vi "Configure Trigger (Pattern).vi"(0 "VISA resource name":refnum<visa-resource-name>, 1 "Pattern Mask (0)":u16, 2 "Edge Source (0: None)":u16(ring) items=["Channel 1"=0, "Channel 2"=1, "Channel 3"=2, "Channel 4"=3, "EXT5"=5, "Digital 0"=7, "Digital 1"=8, "Digital 2"=9, "Digital 3"=10, "Digital 4"=11, "Digital 5"=12, "Digital 6"=13, "Digital 7"=14, "Digital 8"=15, "Digital 9"=16, "Digital 10"=17, "Digital 11"=18, "Digital 12"=19, "Digital 13"=20, "Digital 14"=21, "Digital 15"=22], 3 "Configure Edge (Disable)":bool, 5 "Trigger Source (0: Channel 1)":i32(ring) items=["Channel 1", "Channel 2", "Channel 3", "Channel 4", "EXT", "EXT5", "AC Line", "Digital 0", "Digital 1", "Digital 2", "Digital 3", "Digital 4", "Digital 5", "Digital 6", "Digital 7", "Digital 8", "Digital 9", "Digital 10", "Digital 11", "Digital 12", "Digital 13", "Digital 14", "Digital 15"], 7 "Trigger Level (0.0 V)":dbl, 9 "Pattern Value (0)":u16, 11 "error in (no error)":errorcluster, 12 "EXT Source (0: EXT)":u16(ring) items=["EXT", "EXT5"], 13 "Edge (0: None)":u16(ring) items=["Positive", "Negative"]) -> (4 "VISA resource name out":refnum<visa-resource-name>, 15 "error out":errorcluster)   [LabVIEW 2012, in "RIGOL DS1000 Series.lvlib"]
doc: "Configures pattern trigger settings for an oscilloscope.\n\n<b>Note:</b>\n\nThis VI only applies to the Rigol DS1000B and DS1000D Series models."
uses:
  RIGOL DS1000 Series.lvlib
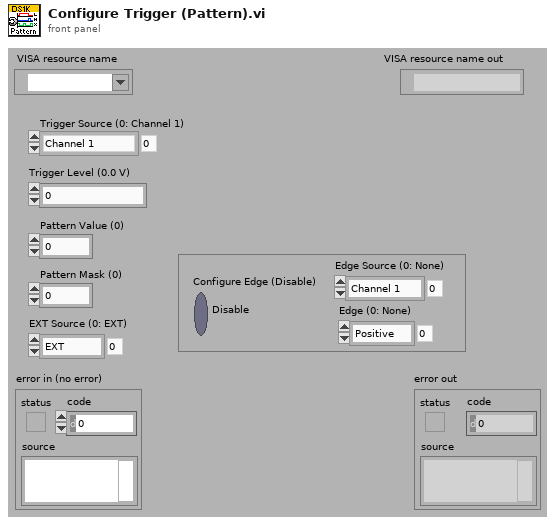
[diagram p1: front panel]
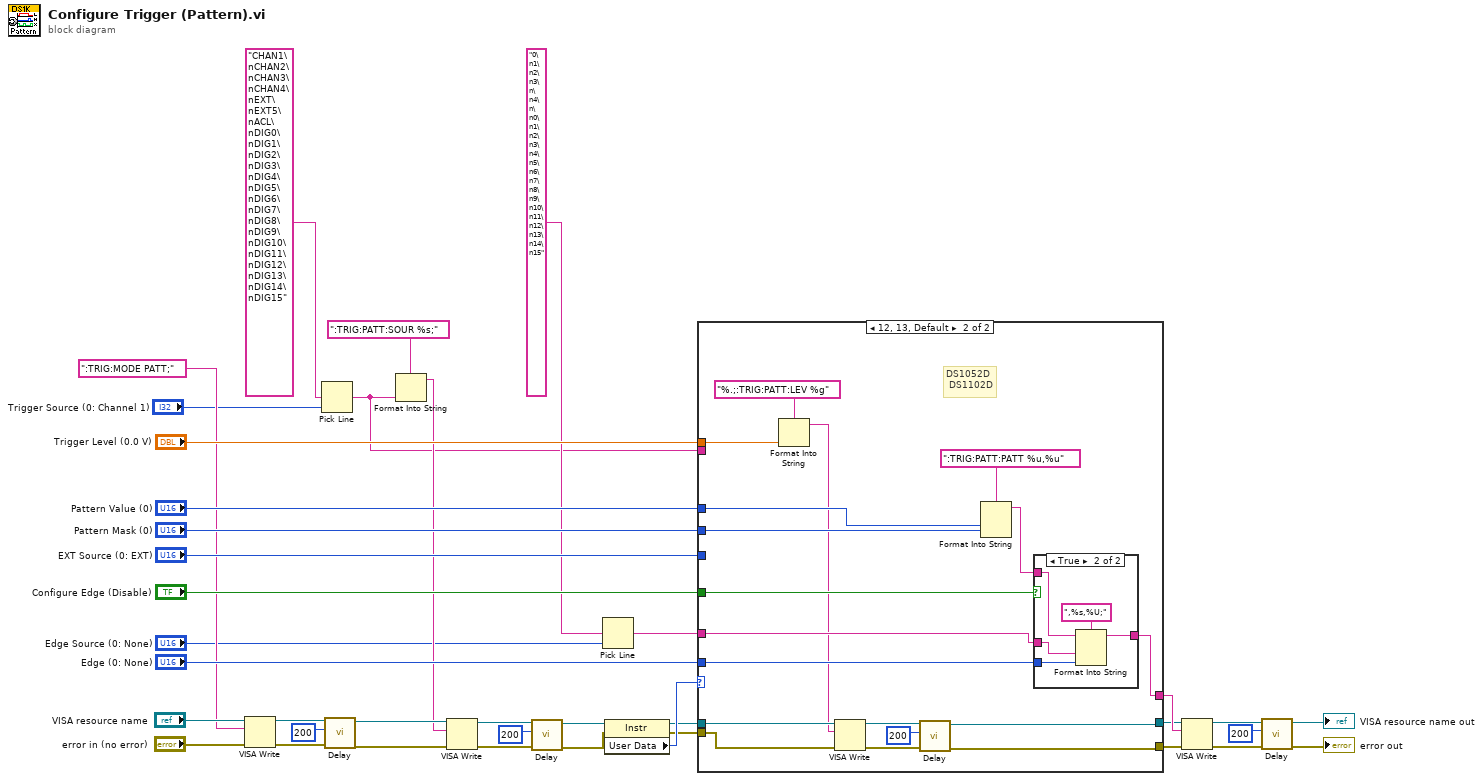
[diagram p0: block diagram]
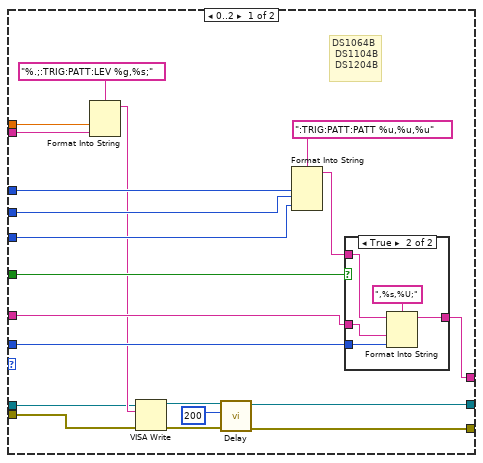
[diagram p2: hidden frame]
diagram:
  n1 = VISA Write(VISA resource name="VISA resource name", write buffer=":TRIG:MODE PATT;" ("Pattern Trigger Type"), error in (no error)="error in (no error)") -> (VISA resource name out=w23:refnum<visa-resource-name>, error out=w24:errorcluster)  [unwired: 1 out]
  n2 = Pick Line(multi-line string="CHAN1\nCHAN2\nCHAN3\nCHAN4\nEXT\nEXT5\nACL\nDIG0\nDIG1\nDIG2\nDIG3\nDIG4\nDIG5\nDIG6\nDIG7\nDIG8\nDIG9\nDIG10\nDIG11\nDIG12\nDIG13\nDIG14\nDIG15" ("多行字符串"), line index="Trigger Source (0: Channel 1)") -> (output string=w1:string)  [unwired: 1 out]
  n3 = call "Delay.vi"("error in (no error)"=w24, "Delay (ms)"=u32 200, "VISA resource name"=w23) -> ("error out"=w14:errorcluster, "VISA resource name out"=w15:refnum<visa-resource-name>)  [unwired: 7 out]
  n4 = Format Into String(format string=":TRIG:PATT:SOUR %s;", w1) -> (resulting string=w13:string)  [unwired: 2 in, 1 out]
  n5 = VISA Write(VISA resource name=w15, write buffer=w13, error in (no error)=w14) -> (VISA resource name out=w17:refnum<visa-resource-name>, error out=w18:errorcluster)  [unwired: 1 out]
  n6 = call "Delay.vi"("error in (no error)"=w18, "Delay (ms)"=u32 200, "VISA resource name"=w17) -> ("error out"=w7:errorcluster, "VISA resource name out"=w8:refnum<visa-resource-name>)  [unwired: 7 out]
  n7 = Pick Line(multi-line string="0\n1\n2\n3\n\n4\n\n0\n1\n2\n3\n4\n5\n6\n7\n8\n9\n10\n11\n12\n13\n14\n15" ("多行字符串"), line index="Edge Source (0: None)") -> (output string=w9:string)  [unwired: 1 out]
  n8 = property class="Instr"(reference=w8, error in=w7) -> (reference out=w5:refnum<visa-resource-name>, error out=w4:errorcluster, "User Data"=w6:u32)
  n9 = case shown="12, 13, Default" w6 {
    tunnel: "Trigger Level (0.0 V)" -> [w58 w82]
    tunnel: "Pattern Value (0)" -> [w55 w79]
    tunnel: "Pattern Mask (0)" -> [w54 w78]
    tunnel: "EXT Source (0: EXT)" -> [w53 _]
    tunnel: "Configure Edge (Disable)" -> [w51 w76]
    tunnel: "Edge (0: None)" -> [w50 w75]
    tunnel: [w49 w74] -> w30
    tunnel: w9 -> [w48 w73]
    tunnel: w5 -> [w43 w69]
    tunnel: w4 -> [w42 w68]
    tunnel: [w41 w66] -> w3
    tunnel: [w40 w65] -> w2
    tunnel: w1 -> [w39 _]
    frame 0..2 {
      # "DS1064B\n DS1104B\n DS1204B"
      n10 = Format Into String(format string="%.;:TRIG:PATT:LEV %g,%s;" ("Trigger Level Command"), w58, w39) -> (resulting string=w44:string)  [unwired: 2 in, 1 out]
      n11 = VISA Write(VISA resource name=w43, write buffer=w44, error in (no error)=w42) -> (VISA resource name out=w46:refnum<visa-resource-name>, error out=w47:errorcluster)  [unwired: 1 out]
      n12 = call "Delay.vi"("error in (no error)"=w47, "Delay (ms)"=u32 200, "VISA resource name"=w46) -> ("error out"=w40:errorcluster, "VISA resource name out"=w41:refnum<visa-resource-name>)  [unwired: 7 out]
      n13 = Format Into String(format string=":TRIG:PATT:PATT %u,%u,%u" ("格式字符串"), w55, w54, w53) -> (resulting string=w52:string)  [unwired: 2 in, 1 out]
      n14 = case shown="True" w51 {
        tunnel: w52 -> [w59 w64]
        tunnel: w48 -> [_ w62]
        tunnel: w50 -> [_ w61]
        tunnel: [w59 w60] -> w49
        frame False {
        }
        frame True {
          n15 = Format Into String(format string=",%s,%U;" ("格式字符串"), initial string=w64, w62, w61) -> (resulting string=w60:string)  [unwired: 1 in, 1 out]
        }
      }
    }
    frame 12, 13, Default {
      # "DS1052D\n DS1102D"
      n16 = Format Into String(format string="%.;:TRIG:PATT:LEV %g" ("Trigger Level Command"), w82) -> (resulting string=w67:string)  [unwired: 2 in, 1 out]
      n17 = VISA Write(VISA resource name=w69, write buffer=w67, error in (no error)=w68) -> (VISA resource name out=w71:refnum<visa-resource-name>, error out=w70:errorcluster)  [unwired: 1 out]
      n18 = call "Delay.vi"("error in (no error)"=w70, "Delay (ms)"=u32 200, "VISA resource name"=w71) -> ("error out"=w65:errorcluster, "VISA resource name out"=w66:refnum<visa-resource-name>)  [unwired: 7 out]
      n19 = Format Into String(format string=":TRIG:PATT:PATT %u,%u" ("格式字符串"), w79, w78) -> (resulting string=w77:string)  [unwired: 2 in, 1 out]
      n20 = case shown="True" w76 {
        tunnel: w77 -> [w83 w88]
        tunnel: w73 -> [_ w86]
        tunnel: w75 -> [_ w85]
        tunnel: [w83 w84] -> w74
        frame False {
        }
        frame True {
          n21 = Format Into String(format string=",%s,%U;" ("格式字符串"), initial string=w88, w86, w85) -> (resulting string=w84:string)  [unwired: 1 in, 1 out]
        }
      }
    }
  }
  n22 = VISA Write(VISA resource name=w3, write buffer=w30, error in (no error)=w2) -> (VISA resource name out=w28:refnum<visa-resource-name>, error out=w27:errorcluster)  [unwired: 1 out]
  n23 = call "Delay.vi"("error in (no error)"=w27, "Delay (ms)"=u32 200, "VISA resource name"=w28) -> ("error out"=→"error out":errorcluster, "VISA resource name out"=→"VISA resource name out":refnum<visa-resource-name>)  [unwired: 7 out]
